vi "Write I2C Slave Address (0).vi"(8 "error in (no error)":errorcluster, 10 "I2C Slave Address (0)":u8=64 format="%.0x", 11 "LINX I2C in":refnum<class "LINX I2C.lvclass">) -> (0 "error out":errorcluster, 3 "LINX I2C out":refnum<class "LINX I2C.lvclass">)   [LabVIEW 2020, in "LINX I2C.lvclass"]
uses:
  LINX I2C.lvclass
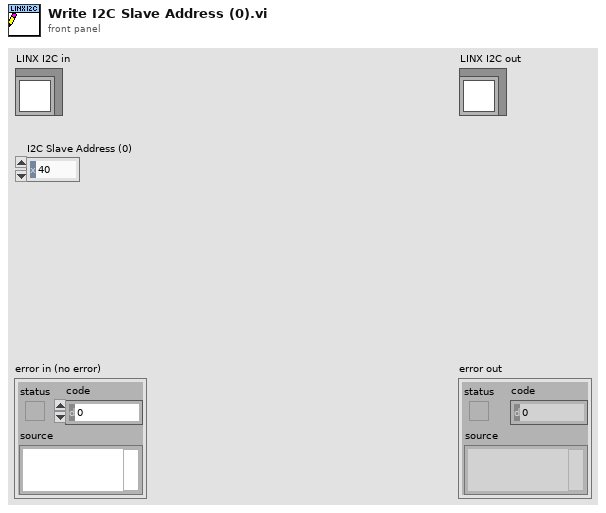
[diagram p1: front panel]
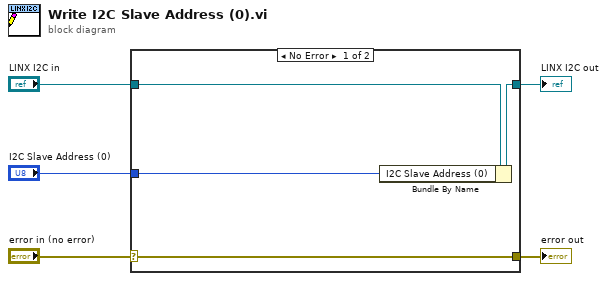
[diagram p0: block diagram]
diagram:
  n1 = case shown="No Error" "error in (no error)" {
    selector: "error in (no error)" -> [w9 w10]
    tunnel: [w9 w10] -> w4
    tunnel: [w7 w11] -> w2
    tunnel: "LINX I2C in" -> [w8 w11]
    tunnel: "I2C Slave Address (0)" -> [w6 _]
    frame No Error {
      n2 = Bundle By Name(cluster=w8, "I2C Slave Address (0)"=w6) -> (w7:refnum<class "LINX I2C.lvclass">)
    }
    frame Error {
    }
  }
  "error out" <- w4
  "LINX I2C out" <- w2
